vi "Result.Read_Write Measurement form CSV File.vi"(8 "error in (no error)":errorcluster, 9 "Read(F)/Write(T)":bool, 10 "Meas In":T1[](array[typedef]) {"Status" items=["LOG", "PASS", "FAIL", "ERROR"]}, 11 "Path":path) -> (0 "error out":errorcluster, 2 "Meas Out":T1[](array[typedef]) {"Status" items=["LOG", "PASS", "FAIL", "ERROR"]}, 3 "Path Dup":path)   [LabVIEW 2024]
uses:
  Result.Measurement Item.ctl
  Result.Measurement and Attribute Item Status.ctl
  Files/File Utils.lvlib
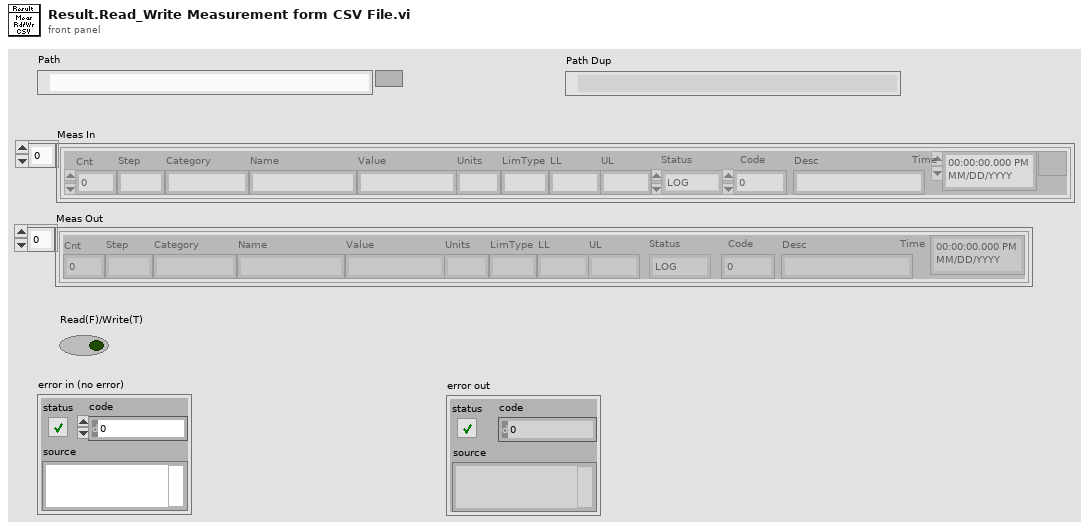
[diagram p1: front panel]
types:
  T1 = typedef "Result.Measurement Item.ctl" = cluster{"Cnt":i32, "Step":string, "Category":string, "Name":string, "Value":string, "Units":string, "LimType":string, "LL":string, "UL":string, "Status":T2, "Code":i32, "Desc":string, "Time":timestamp}
  T2 = typedef "Result.Measurement and Attribute Item Status.ctl" = i32
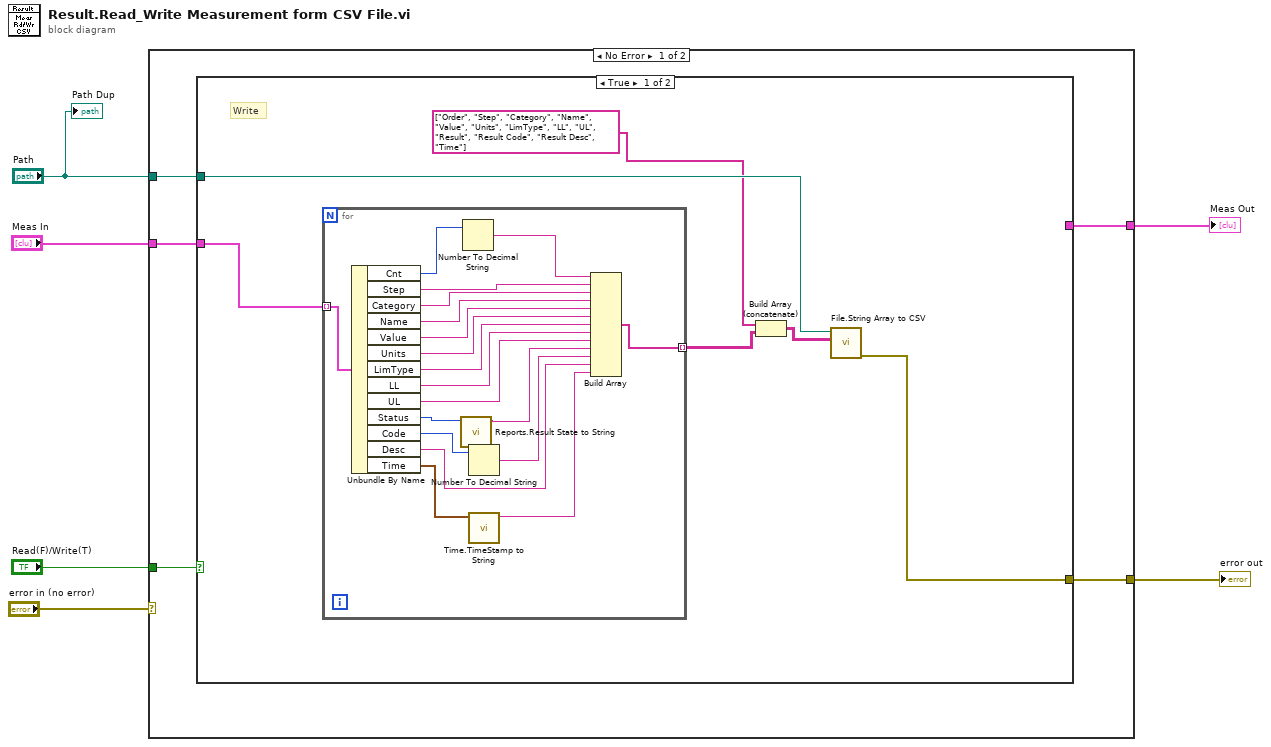
[diagram p0: block diagram]
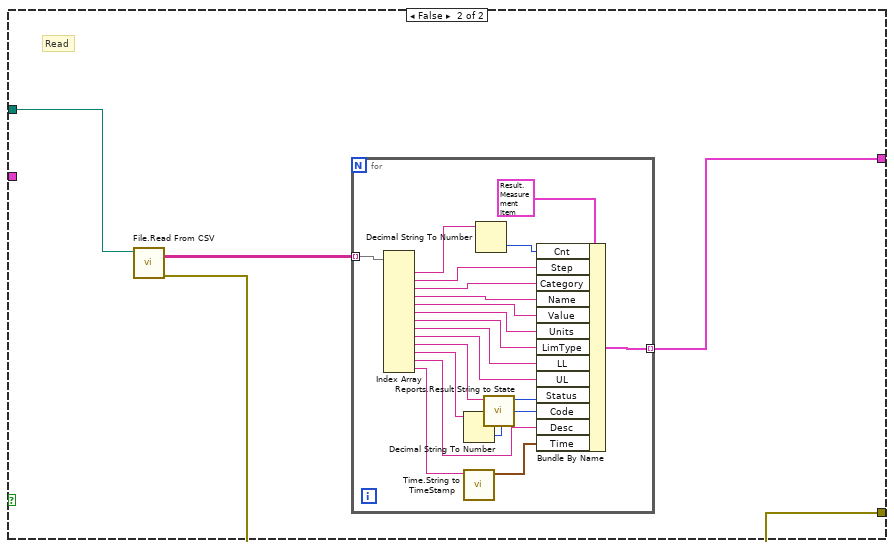
[diagram p2: hidden frame]
diagram:
  n1 = case shown="No Error" "error in (no error)" {
    selector: "error in (no error)" -> [_ w61]
    tunnel: "Read(F)/Write(T)" -> [w11 _]
    tunnel: "Path" -> [w10 _]
    tunnel: "Meas In" -> [w9 _]
    tunnel: [w8 w61] -> w3
    tunnel: [w7 _] -> w1
    frame No Error {
      n2 = case shown="True" w11 {
        tunnel: w10 -> [w16 w40]
        tunnel: w9 -> [w17 _]
        tunnel: [w15 w38] -> w8
        tunnel: [_ w37] -> w7
        frame True {
          # "Write"
          n3 = for {
            tunnel: w17 -> [w36] mode=indexing
            tunnel: [w22] -> w12 mode=indexing
            n4 = Unbundle By Name(w36) -> ("Cnt"=w35:i32, "Step"=w32:string, "Category"=w31:string, "Name"=w30:string, "Value"=w29:string, "Units"=w28:string, "LimType"=w27:string, "LL"=w26:string, "UL"=w25:string, "Status"=w21:T2, "Code"=w34:i32, "Desc"=w23:string, "Time"=w19:timestamp)
            n5 = call "Reports.Result State to String.vi"("Result State"=w21) -> ("String Out"=w20:string)  [unwired: 6 in]
            n6 = Number To Decimal String(number=w35) -> (decimal integer string=w33:string)  [unwired: 1 in]
            n7 = Number To Decimal String(number=w34) -> (decimal integer string=w24:string)  [unwired: 1 in]
            n8 = call "Time.TimeStamp to String.vi"("Time Stamp in"=w19) -> ("Time String Out"=w18:string)  [unwired: 10 in]
            n9 = Build Array(w33, w32, w31, w30, w29, w28, w27, w26, w25, w20, w24, w23, w18) -> (w22:string[])
          }
          n10 = Build Array (concatenate)(string[] ["Order", "Step", "Category", "Name", "Value", "Units", "LimType", "LL", "UL", "Result", "Result Code", "Result Desc", "Time"], w12) -> (w14:string[][])
          n11 = call "File.String Array to CSV.vi"("2D Str"=w14, "FilePath"=w16) -> ("Error Out"=w15:errorcluster)  [unwired: 8 in, 1 out]
        }
        frame False {
          # "Read"
          n12 = call "File.Read From CSV.vi"("File"=w40) -> ("error out"=w38:errorcluster, "Data"=w39:string[][])  [unwired: 8 in, 1 out]
          n13 = for {
            tunnel: w39 -> [w59] mode=indexing
            tunnel: [w41] -> w37 mode=indexing
            n14 = Index Array(array=w59) -> (element #1=w58:string, element #2=w56:string, element #3=w55:string, element #4=w54:string, element #5=w53:string, element #6=w52:string, element #7=w51:string, element #8=w50:string, element #9=w49:string, element #10=w48:string, element #11=w46:string, element #12=w44:string, element #13=w42:string)  [unwired: 13 in]
            n15 = Decimal String To Number(string=w46) -> (number=w45:i32)  [unwired: 2 in, 1 out]
            n16 = call "Time.String to TimeStamp.vi"("Time String In"=w42) -> ("Time Stamp Out"=w43:timestamp)  [unwired: 10 in]
            n17 = Decimal String To Number(string=w58) -> (number=w57:i32)  [unwired: 2 in, 1 out]
            n18 = call "Reports.Result String to State.vi"("State String"=w48) -> ("Result State"=w47:T2)  [unwired: 6 in]
            n19 = Bundle By Name(cluster=T1 {"Cnt"=0, "Step"="", "Category"="", "Name"="", "Value"="", "Units"="", "LimType"="", "LL"="", "UL"="", "Status"=0, "Code"=0, "Desc"="", "Time"=timestamp(0 s since 1904-01-01)} ("Meas"), "Cnt"=w57, "Step"=w56, "Category"=w55, "Name"=w54, "Value"=w53, "Units"=w52, "LimType"=w51, "LL"=w50, "UL"=w49, "Status"=w47, "Code"=w45, "Desc"=w44, "Time"=w43) -> (w41:T1)
          }
        }
      }
    }
    frame Error {
    }
  }
  "Meas Out" <- w1
  "error out" <- w3
  "Path Dup" <- "Path"
